vi "air_mass_flow_calculate.vi"(8 "input signal":dbl) -> (3 "output signal":dbl)   [LabVIEW 2014]
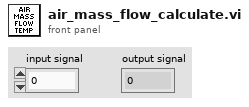
[diagram p1: front panel]
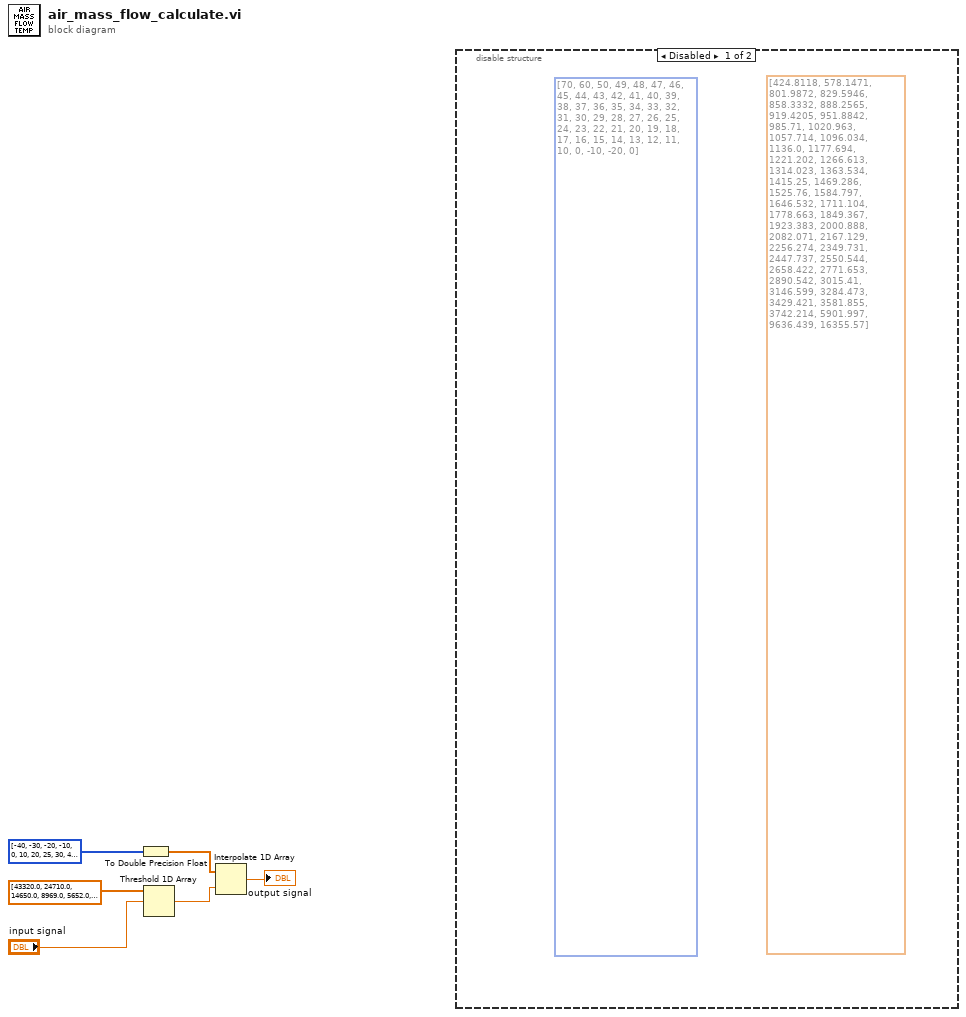
[diagram p0: block diagram]
diagram:
  n1 = To Double Precision Float(number=i32[] [-40, -30, -20, -10, 0, 10, 20, 25, 30, 40, 50, 60, 70, 80, 90, 100, 110, 120, 130, 140, 150]) -> (double precision float=w4:dbl[])
  n2 = Threshold 1D Array(2:"input signal", 3:dbl[] [43320.0, 24710.0, 14650.0, 8969.0, 5652.0, 3663.0, 2433.0, 2000.0, 1653.0, 1148.0, 813.0, 587.0, 431.0, 321.0, 243.0, 186.0, 144.0, 113.0, 90.0, 72.0, 58.0] ("array of numbers or points")) -> (0:w5:dbl)  [unwired: 1 in]
  n3 = Interpolate 1D Array(1:w5, 2:w4) -> (0:→"output signal":dbl)
  n4 = disable-structure shown="Disabled" {
    frame Disabled {
      (unwired) dbl[] [424.8118, 578.1471, 801.9872, 829.5946, 858.3332, 888.2565, 919.4205, 951.8842, 985.71, 1020.963, 1057.714, 1096.034, 1136.0, 1177.694, 1221.202, 1266.613, 1314.023, 1363.534, 1415.25, 1469.286, 1525.76, 1584.797, 1646.532, 1711.104, 1778.663, 1849.367, 1923.383, 2000.888, 2082.071, 2167.129, 2256.274, 2349.731, 2447.737, 2550.544, 2658.422, 2771.653, 2890.542, 3015.41, 3146.599, 3284.473, 3429.421, 3581.855, 3742.214, 5901.997, 9636.439, 16355.57]
      (unwired) i32[] [70, 60, 50, 49, 48, 47, 46, 45, 44, 43, 42, 41, 40, 39, 38, 37, 36, 35, 34, 33, 32, 31, 30, 29, 28, 27, 26, 25, 24, 23, 22, 21, 20, 19, 18, 17, 16, 15, 14, 13, 12, 11, 10, 0, -10, -20, 0]
    }
    frame Enabled {
    }
  }
